vi "SLIT_TRANS_Read_Config.vi"(4 "error in (no error)":errorcluster, 7 "Config Refnum":T1) -> (0 "error out":errorcluster, 2 "All Found?":bool, 3 "refnum out":T1)   [LabVIEW 2015]
uses:
  <vilib>/Utility/config.llb/Config Data RefNum.ctl
  <vilib>/Utility/config.llb/Read Key (I32).vi
  GSP_SLIT_Global.vi
  <vilib>/Utility/config.llb/NI_LVConfig.lvlib
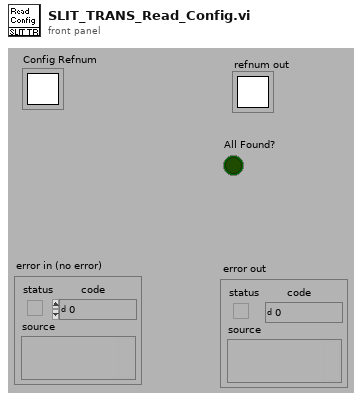
[diagram p1: front panel]
types:
  T1 = typedef "NI_LVConfig.lvlib/Config Data RefNum.ctl" = refnum<k1>
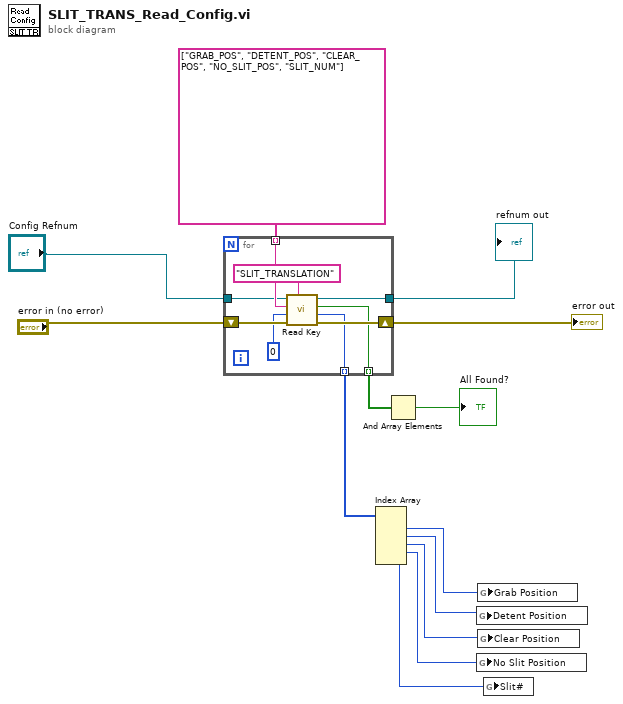
[diagram p0: block diagram]
diagram:
  n1 = for {
    shift-right: [w20] -> w9
    shift-left: "error in (no error)" -> [w22]
    tunnel: [w19] -> w10
    tunnel: string[] ["GRAB_POS", "DETENT_POS", "CLEAR_POS", "NO_SLIT_POS", "SLIT_NUM"] -> [w18] mode=indexing
    tunnel: "Config Refnum" -> [w17]
    tunnel: [w15] -> w8 mode=indexing
    tunnel: [w14] -> w7 mode=indexing
    n2 = call-poly <vilib>:"Read Key.vi"("section"="SLIT_TRANSLATION", "error in (no error)"=w22, "default value"=0, "key"=w18, "refnum"=w17) -> ("error out"=w20:errorcluster, "value"=w15:i32, "found?"=w14:bool, "refnum out"=w19:T1)  [unwired: 3 in]
  }
  "error out" <- w9
  "refnum out" <- w10
  n3 = Index Array(array=w8) -> (element #1=w5:i32, element #2=w4:i32, element #3=w3:i32, element #4=w2:i32, element #5=w1:i32)  [unwired: 5 in]
  n4 = And Array Elements(Boolean array=w7) -> (logical AND=→"All Found?":bool)
  n5 = global write "GSP_SLIT_Global.vi" "Detent Position"(w4) -> ()
  n6 = global write "GSP_SLIT_Global.vi" "No Slit Position"(w2) -> ()
  n7 = global write "GSP_SLIT_Global.vi" "Grab Position"(w5) -> ()
  n8 = global write "GSP_SLIT_Global.vi" "Clear Position"(w3) -> ()
  n9 = global write "GSP_SLIT_Global.vi" "Slit#"(w1) -> ()
